vi "temperature_indicator.vi"() -> ()   [LabVIEW 2016]
uses:
  <vilib>/LabVIEW Interface for Arduino/Type Defs/Board Type.ctl
  <vilib>/LabVIEW Interface for Arduino/Type Defs/Connection Type.ctl
  <vilib>/LabVIEW Interface for Arduino/Type Defs/Pin Mode.ctl
  <vilib>/LabVIEW Interface for Arduino/LabVIEW Interface for Arduino.lvlib
panel:
  in  "Third threshold":dbl
  in  "Second threshold":dbl
  in  "First threshold":dbl
  out "Third Level":bool
  out "Second Level":bool
  out "First Level":bool
  out "Thermometer":dbl(slide) scale=0.0..100.0
  in  "stop":bool
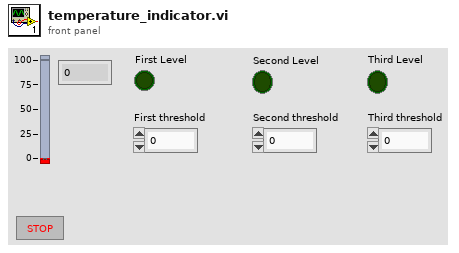
[diagram p1: front panel]
types:
  T1 = typedef "LabVIEW Interface for Arduino.lvlib/Connection Type.ctl" = enum8{"USB / Serial", "XBEE", "BlueSmirf (Bluetooth)"}
  T2 = typedef "LabVIEW Interface for Arduino.lvlib/Board Type.ctl" = enum16{"Uno", "Dimuelanove w/Atmega 328", "Mega 2560"}
  T3 = typedef "LabVIEW Interface for Arduino.lvlib/Arduino Resource.ctl" = cluster{"VISA resource":refnum<visa-resource-name>, "Board Type":T2, "Connection Type":enum8{"USB / Serial"}, "Bytes Per Packet (15)":u8}
  T4 = typedef "LabVIEW Interface for Arduino.lvlib/Pin Mode.ctl" = enum8{"Input", "Output"}
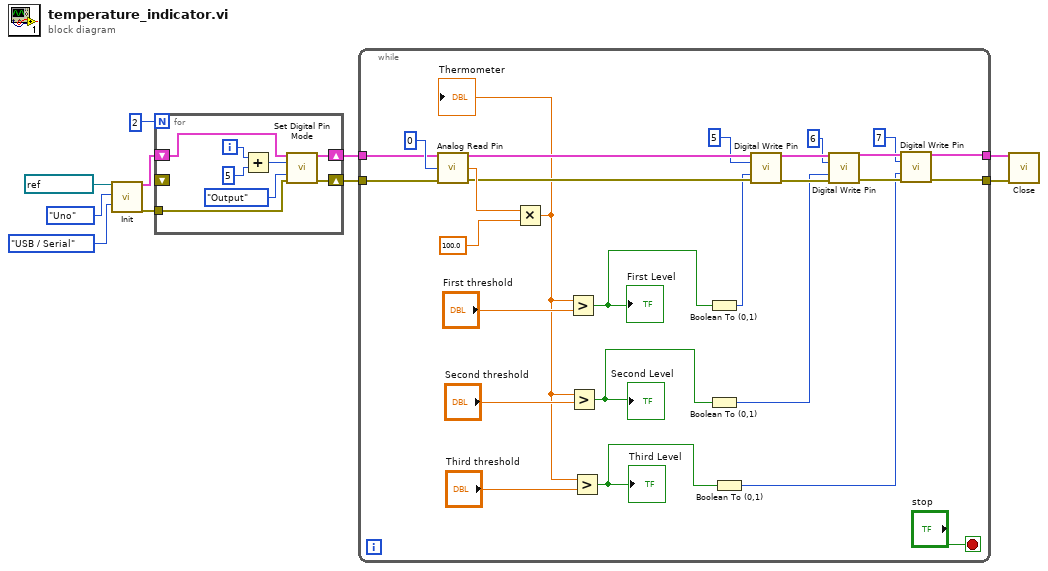
[diagram p0: block diagram]
diagram:
  n1 = call <vilib>:"Init.vi"("VISA resource"=refnum<visa-resource-name> "COM3", "Board Type (Uno)"=Board_Type."Uno", "Connection Type (USB/Serial)"=Connection_Type."USB / Serial") -> ("Arduino Resource"=w3:T3, "error out"=w6:errorcluster)  [unwired: 15 in]
  n2 = for {
    N: 2 -> [_]
    tunnel: w6 -> [w16]
    shift-right: [w13] -> w5
    shift-left: w3 -> [w11]
    shift-right: [w12] -> w4
    shift-left: _ -> [_]
    i -> [w18]
    n3 = Add(x=w18, y=5) -> (x+y=w15:i32)
    n4 = call <vilib>:"Set Digital Pin Mode.vi"("Arduino Resource"=w11, "Digital I/O Pin"=w15, "Pin Mode (Input)"=Pin_Mode."Output", "error in"=w16) -> ("Arduino Resource"=w13:T3, "error out"=w12:errorcluster)  [unwired: 10 in]
  }
  n5 = while {
    tunnel: [w35] -> w2
    tunnel: w5 -> [w43]
    tunnel: w4 -> [w42]
    tunnel: [w34] -> w1
    stop <- "stop" stop-if-true
    n6 = call <vilib>:"Analog Read Pin.vi"("Arduino Resource"=w43, "Analog Input Pin (0)"=u8 0, "error in"=w42) -> ("Arduino Resource"=w33:T3, "Voltage"=w41:dbl, "error out"=w32:errorcluster)  [unwired: 10 in]
    n7 = Multiply(x=w41, y=100.0) -> (x*y=w25:dbl)
    "Thermometer" <- w25
    n8 = Greater?(x=w25, y="First threshold") -> (0:w24:bool)
    "First Level" <- w24
    n9 = Greater?(x=w25, y="Second threshold") -> (0:w22:bool)
    "Second Level" <- w22
    n10 = Greater?(x=w25, y="Third threshold") -> (0:w21:bool)
    "Third Level" <- w21
    n11 = Boolean To (0,1)(Boolean=w24) -> (0, 1=w23:i16)
    n12 = Boolean To (0,1)(Boolean=w22) -> (0, 1=w20:i16)
    n13 = Boolean To (0,1)(Boolean=w21) -> (0, 1=w19:i16)
    n14 = call <vilib>:"Digital Write Pin.vi"("Arduino Resource"=w33, "Digital I/O Pin (0)"=u8 5, "Value (0)"=w23, "error in"=w32) -> ("Arduino Resource"=w39:T3, "error out"=w37:errorcluster)  [unwired: 10 in]
    n15 = call <vilib>:"Digital Write Pin.vi"("Arduino Resource"=w39, "Digital I/O Pin (0)"=u8 6, "Value (0)"=w20, "error in"=w37) -> ("Arduino Resource"=w38:T3, "error out"=w36:errorcluster)  [unwired: 10 in]
    n16 = call <vilib>:"Digital Write Pin.vi"("Arduino Resource"=w38, "Digital I/O Pin (0)"=u8 7, "Value (0)"=w19, "error in"=w36) -> ("Arduino Resource"=w35:T3, "error out"=w34:errorcluster)  [unwired: 10 in]
  }
  n17 = call <vilib>:"Close.vi"("Arduino Resource"=w2, "error in"=w1) -> ()  [unwired: 13 in, 1 out]
